vi "Raster.vi"(10 "Pixel Data in":u32[][](array[numeric]), 11 "Scene in":refnum<class "Scene.lvclass">) -> (2 "Pixel Data out":u32[][](array[numeric]), 3 "Scene out":refnum<class "Scene.lvclass">)   [LabVIEW 2022 SP3, in "Application.lvlib" / "Scene.lvclass"]
uses:
  Scene.lvclass
  Scene.lvclass/Scene.ctl
  edb3f0c2-b950-4a44-8897-096d76b30880.vi
  76d78098-f527-454b-a08a-aac5a717328f.vi
  <vilib>/Utility/High Resolution Relative Seconds.vi
  Libraries/3D/Convert Point 2D (SGL) to Point 2D (I32).vi
  Libraries/Raster/Draw Triangle.vi
  Libraries/Raster/Draw Filled Triangle.vi
  Libraries/Raster/Clear Framebuffer.vi
  Libraries/Raster/Draw Line.vi
  Libraries/Raster/Draw Flat Bottom Filled Triangle.vi
  Libraries/Raster/Sort Points.vi
  Libraries/Raster/Draw Flat Top Filled Triangle.vi
  Libraries/Raster/Draw Line.vi/ce09c930-e75c-45b5-9de7-7d3097d91b09.vi
  Libraries/Raster/Draw Line.vi/8aa8c736-0805-475e-bbf3-9937bbefdeb4.vi
  Libraries/Raster/Draw Horizontal Line.vi
  Libraries/Raster/Draw Flat Bottom Filled Triangle.vi/c0c82237-b583-4fc1-b44f-40d02a28ecfd.vi
  Libraries/Raster/Draw Flat Bottom Filled Triangle.vi/53435b12-820c-4aea-aec4-7de16a894549.vi
  <userlib>/_OpenG.lib/array/array.llb/Sort Array__ogtk.vi
  <userlib>/_OpenG.lib/array/array.llb/Sort 1D Array (I32)__ogtk.vi
  <vilib>/Utility/colorconv.llb/Color to RGB.vi
  <vilib>/Utility/colorconv.llb/RGB to Color.vi
  Libraries/3D/3D.lvlib
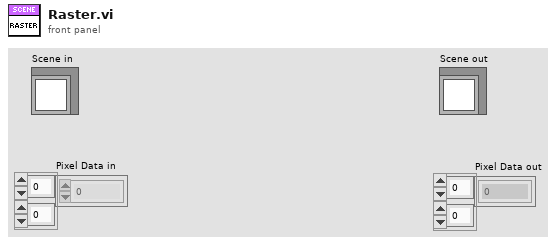
[diagram p1: front panel]
types:
  T1 = typedef "3D.lvlib/Triangle 2D.ctl" = cluster{"Point 1":T2, "Point 2":T2, "Point 3":T2, "Fill Colour":u32, "Alpha":dbl, "Alpha Blending Enabled":bool}
  T2 = typedef "3D.lvlib/Point 2D.ctl" = cluster{"x":sgl, "y":sgl}
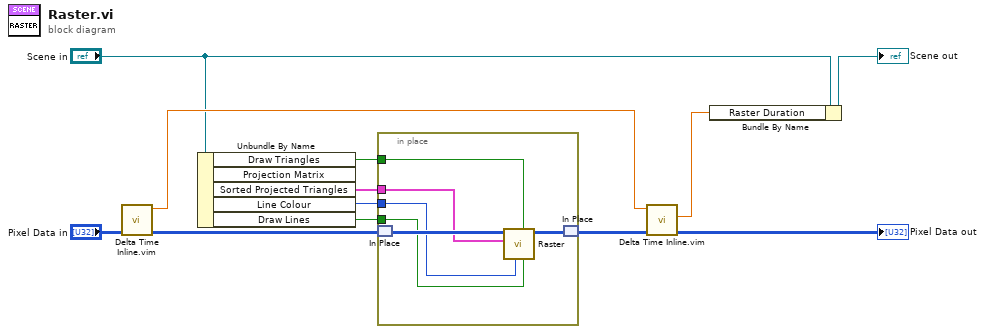
[diagram p0: block diagram]
diagram:
  n1 = call "Delta Time Inline.vim"("value in"="Pixel Data in") -> ("value out"=w8:u32[][], "Relative Seconds out [s]"=w12:dbl)  [unwired: 8 in, 1 out]
  n2 = Unbundle By Name("Scene in") -> ("Draw Triangles"=w3:bool, "Sorted Projected Triangles"=w7:T1[], "Line Colour"=w2:u32, "Draw Lines"=w1:bool)  [unwired: 1 out]
  n3 = in-place {
    in-place-border: w7 -> [w16]
    in-place-border: w3 -> [w15]
    in-place-border: w2 -> [w14]
    in-place-border: w1 -> [w13]
    n4 = in-place-match #1(w8) -> (w18:u32[][])
    n5 = call "Raster.vi"("Draw Lines"=w13, "Draw Triangles"=w15, "Line Colour"=w14, "Triangles Sorted"=w16, "Pixel Data in"=w18) -> ("Pixel Data out"=w17:u32[][])  [unwired: 6 in]
    n6 = in-place-match #1(w17) -> (w11:u32[][])
  }
  n7 = call "Delta Time Inline.vim"("value in"=w11, "Relative Seconds in [s]"=w12) -> ("value out"=→"Pixel Data out":u32[][], "Delta Time [s]"=w4:dbl)  [unwired: 7 in, 1 out]
  n8 = Bundle By Name(cluster="Scene in", "Raster Duration"=w4) -> (→"Scene out":refnum<class "Scene.lvclass">)
